vi "SACB.vi"(6 "timeout":i32=50, 7 "Command":enum16{"Create", "Read", "Close"}(ring), 8 "Error In":errorcluster, 11 "Model Name":T1) -> (0 "Error Out":errorcluster, 2 "Connected?":bool, 3 "Digital Inputs":T2)   [LabVIEW 2017]
uses:
  controls/SACB DI.ctl
  controls/Model Name.ctl
  <vilib>/Modbus/master/Modbus Master.lvclass
  <vilib>/Modbus/master/Create Master Instance (TCP).vi
panel:
  out "register values":u16[][](array[numeric])
  # "RS_Clamping_top_Front\nRS_Clamping_bottom_Front\nRS_Clamping_MotorLH_Front\nRS_Clamping_MotorRH_Front\nIPS_Part presence_top_LH\nIPS_Part presence_Bottom_LH\nIPS_Part presence_top_RH\nIPS_Part presence_Bottom_RH\nIPS_Load engaged_1\nIPS_Part presence_2\nIPS_Load engaged_MCO_LH\nIPS_Load engaged_MCO_RH"
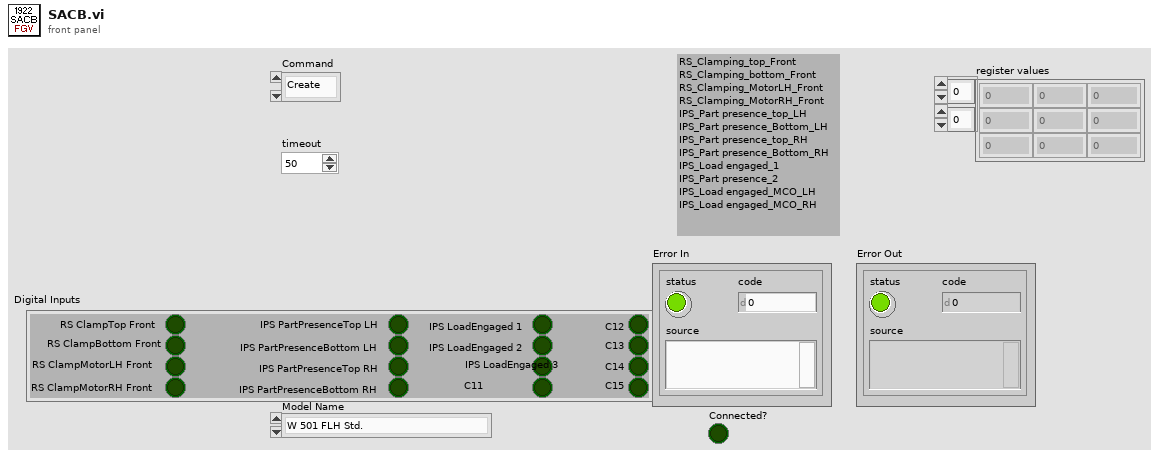
[diagram p1: front panel]
types:
  T1 = typedef "Model Name.ctl" = enum16{"W 501 FLH Std.", "W 501 FRH Std.", "W 601 FR RH Std", "W 601 FR LH Std", "W 601 RR RH Std", "W 601 RR LH Std", "W 601 FR RH AP", "W 601 FR LH AP", "W 601 RR RH AP", "W 601 RR LH AP"}
  T2 = typedef "SACB DI.ctl" = cluster{"RS ClampTop Front":bool, "RS ClampBottom Front":bool, "RS ClampMotorLH Front":bool, "RS ClampMotorRH Front":bool, "IPS PartPresenceTop LH":bool, "IPS PartPresenceBottom LH":bool, "IPS PartPresenceTop RH":bool, "IPS PartPresenceBottom RH":bool, "IPS LoadEngaged 1":bool, "IPS LoadEngaged 2":bool, "IPS LoadEngaged 3":bool, "C11":bool, "C12":bool, "C13":bool, "C14":bool, "C15":bool}
  T3 = cluster{"[0]":bool, "[1]":bool, "[2]":bool, "[3]":bool, "[4]":bool, "[5]":bool, "[6]":bool, "[7]":bool, "[8]":bool, "[9]":bool, "[10]":bool, "[11]":bool, "[12]":bool, "[13]":bool, "[14]":bool, "[15]":bool}
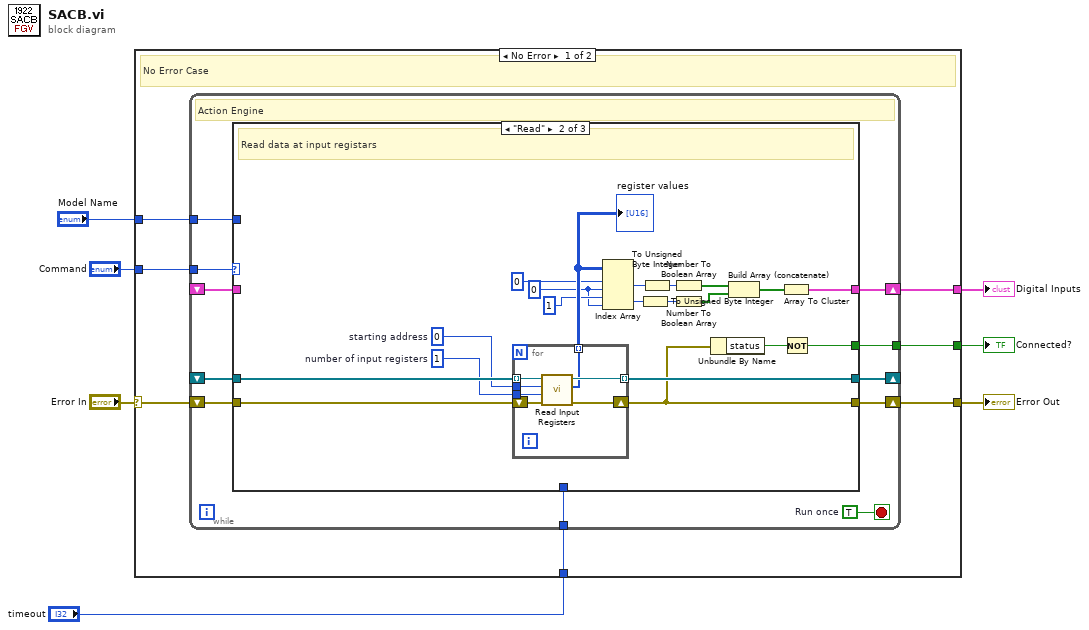
[diagram p0: block diagram]
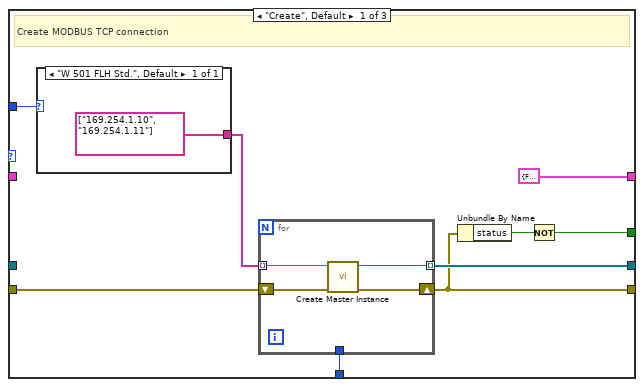
[diagram p2: hidden frame]
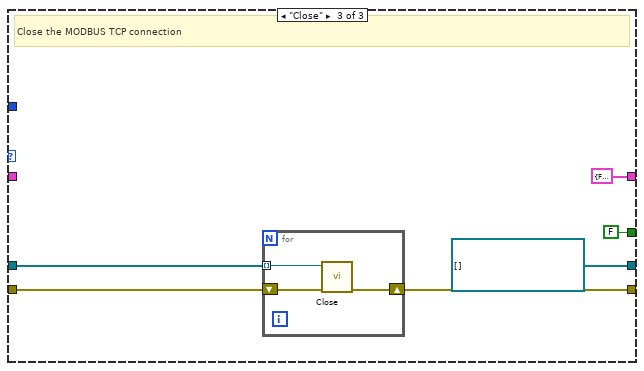
[diagram p3: hidden frame]
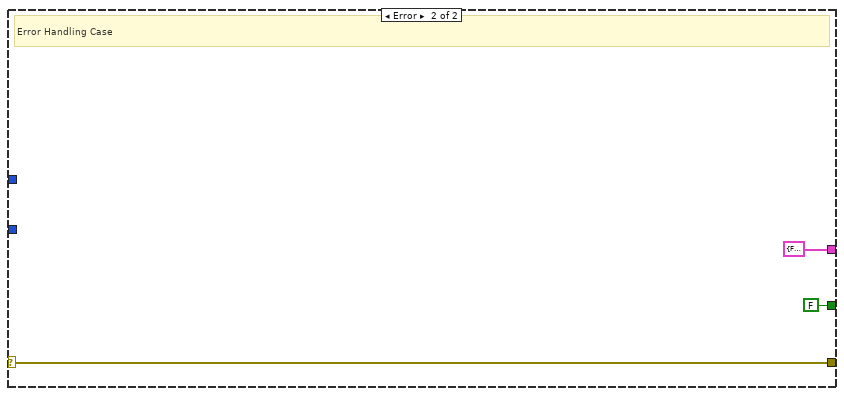
[diagram p4: hidden frame]
diagram:
  n1 = case shown="No Error" "Error In" {
    selector: "Error In" -> [w13 w78]
    tunnel: [w14 w78] -> w6
    tunnel: "Command" -> [w12 _]
    tunnel: [w11 T3 {"[0]"=FALSE, "[1]"=FALSE, "[2]"=FALSE, "[3]"=FALSE, "[4]"=FALSE, "[5]"=FALSE, "[6]"=FALSE, "[7]"=FALSE, "[8]"=FALSE, "[9]"=FALSE, "[10]"=FALSE, "[11]"=FALSE, "[12]"=FALSE, "[13]"=FALSE, "[14]"=FALSE, "[15]"=FALSE}] -> w4
    tunnel: "Model Name" -> [w10 _]
    tunnel: [w9 FALSE] -> w2
    tunnel: "timeout" -> [w8 _]
    frame No Error {
      # "No Error Case"
      n2 = while {
        tunnel: w12 -> [w23]
        shift-right: [w25] -> w14
        shift-left: w13 -> [w24]
        shift-right: [w21] -> _
        shift-left: _ -> [w20]
        shift-right: [w19] -> w11
        shift-left: _ -> [w18]
        tunnel: w10 -> [w17]
        tunnel: [w16] -> w9
        tunnel: w8 -> [w15]
        stop <- w22 stop-if-true
        w22 = TRUE  # Run once
        # "Action Engine"
        n3 = case shown="\"Read\"" w23 {
          tunnel: [w29 w45 w71] -> w25
          tunnel: w24 -> [w34 w59 w72]
          tunnel: [w33 w58 refnum<class "Modbus Master.lvclass">[] []] -> w21
          tunnel: w20 -> [_ w57 w70]
          tunnel: [T3 {"[0]"=FALSE, "[1]"=FALSE, "[2]"=FALSE, "[3]"=FALSE, "[4]"=FALSE, "[5]"=FALSE, "[6]"=FALSE, "[7]"=FALSE, "[8]"=FALSE, "[9]"=FALSE, "[10]"=FALSE, "[11]"=FALSE, "[12]"=FALSE, "[13]"=FALSE, "[14]"=FALSE, "[15]"=FALSE} w47 T3 {"[0]"=FALSE, "[1]"=FALSE, "[2]"=FALSE, "[3]"=FALSE, "[4]"=FALSE, "[5]"=FALSE, "[6]"=FALSE, "[7]"=FALSE, "[8]"=FALSE, "[9]"=FALSE, "[10]"=FALSE, "[11]"=FALSE, "[12]"=FALSE, "[13]"=FALSE, "[14]"=FALSE, "[15]"=FALSE}] -> w19
          tunnel: w18 -> [_ _ _]
          tunnel: w17 -> [w32 _ _]
          tunnel: [w27 w44 FALSE] -> w16
          tunnel: w15 -> [w26 _ _]
          frame "Create", Default {
            # "Create MODBUS TCP connection"
            n4 = case shown="\"W 501 FLH Std.\", Default" w32 {
              tunnel: [string[] ["169.254.1.10", "169.254.1.11"]] -> w31
              frame "W 501 FLH Std.", Default {
              }
            }
            n5 = for {
              tunnel: [w36] -> w33 mode=indexing
              shift-right: [w38] -> w29
              shift-left: w34 -> [w37]
              tunnel: w31 -> [w35] mode=indexing
              tunnel: w26 -> [_]
              n6 = call-poly <vilib>:"Create Master Instance.vi"("error in (no error)"=w37, "address"=w35) -> ("error out"=w38:errorcluster, "TCP master instance"=w36:refnum<class "Modbus Master.lvclass">)  [unwired: 8 in]
            }
            n7 = Unbundle By Name(w29) -> ("status"=w28:bool)
            n8 = Not(x=w28) -> (.not. x?=w27:bool)
          }
          frame "Read" {
            w42 = 0 ("disabled index (col)")
            w55 = u16 1  # number of input registers
            w56 = u16 0  # starting address
            # "Read data at input registars"
            n9 = for {
              tunnel: [w64] -> w58 mode=indexing
              tunnel: w57 -> [w63] mode=indexing
              tunnel: w56 -> [w62]
              tunnel: w55 -> [w61]
              tunnel: [w60] -> w52 mode=indexing
              shift-right: [w65] -> w45
              shift-left: w59 -> [w66]
              n10 = call-dynamic "Read Input Registers.vi"("error in (no error)"=w66, "number of input registers"=w61, "starting address"=w62, "Modbus master in"=w63) -> ("error out"=w65:errorcluster, "register values"=w60:u16[], "Modbus master out"=w64:refnum<class "Modbus Master.lvclass">)  [unwired: 5 in]
            }
            "register values" <- w52
            n11 = Index Array(array=w52, index (row) #1=0 ("index"), index (col) #1=w42, index (row) #2=1 ("disabled index (col)"), index (col) #2=w42) -> (element #1=w53:u16, element #2=w50:u16)
            n12 = To Unsigned Byte Integer(number=w50) -> (unsigned 8bit integer=w40:u8)
            n13 = To Unsigned Byte Integer(number=w53) -> (unsigned 8bit integer=w41:u8)
            n14 = Number To Boolean Array(number=w41) -> (Boolean array=w54:bool[])
            n15 = Number To Boolean Array(number=w40) -> (Boolean array=w48:bool[])
            n16 = Unbundle By Name(w45) -> ("status"=w46:bool)
            n17 = Build Array (concatenate)(w54, w48) -> (w49:bool[])
            n18 = Array To Cluster(array=w49) -> (cluster=w47:T3)
            n19 = Not(x=w46) -> (.not. x?=w44:bool)
          }
          frame "Close" {
            # "Close the MODBUS TCP connection"
            n20 = for {
              tunnel: w70 -> [w73] mode=indexing
              shift-right: [w74] -> w71
              shift-left: w72 -> [w75]
              n21 = call-dynamic "Close.vi"("error in (no error)"=w75, "Modbus master in"=w73) -> ("error out"=w74:errorcluster)  [unwired: 9 in]
            }
          }
        }
      }
    }
    frame Error {
      # "Error Handling Case"
    }
  }
  "Error Out" <- w6
  "Digital Inputs" <- w4
  "Connected?" <- w2
